vi "spotfindsettingsIngoHeucke.vi"(7 "Enum":T3(ring)=enum."change", 9 "already x spots found":i16=46, 11 "notes 2":refnum<vi>) -> (0 "settings":string="\n43 spot(s) found\nclose filter:  TRUE\nconnectivity 4/8: TRUE\nthreshold (min):  25\nthreshold (max):  1000\nselection values:\nParameter: Area (pixels)\n\t lower value: 16.00\n\t upper value: 245.00\n\t include: TRUE\nParameter: Heywood circularity factor\n\t lower value: 0.95\n\t upper value: 1.53\n\t include: TRUE\n", 2 "spotfinding settings":T2={"show all"=FALSE, "threshold/morph"=FALSE, "particle filter"=FALSE, "spot marks"=FALSE, "close filter"=TRUE, "connectivity 4/8"=TRUE, "range"={"Lower value"=25.0, "Upper value"=1000.0}, "PSF-size"=5, "Parameters"=[{"Parameter"=enum."Area (pixels)", "Lower Value"=16.0, "Upper Value"=245.0, "Interval"=TRUE}, {"Parameter"=enum."Heywood circularity factor", "Lower Value"=0.95, "Upper Value"=1.53, "Interval"=TRUE}]} {"range"."Upper value" format="%.2f"; "range"."Lower value" format="%.2f"; "Parameters"."Upper Value" format="%.2f"; "Parameters"."Lower Value" format="%.2f"}, 4 "coordinates":i32[][](array[numeric])=[[93, 0, 103, 10], [389, 8, 399, 18], [260, 10, 270, 20], [132, 13, 142, 23], [298, 19, 308, 29], [338, 32, 348, 42], [210, 38, 220, 48], [81, 41, 91, 51], [377, 45, 387, 55], [249, 50, 259, 60], [290, 60, 300, 70], [329, 74, 339, 84], [237, 89, 247, 99], [315, 110, 325, 120], [188, 117, 198, 127], [355, 124, 365, 134], [225, 128, 235, 138], [98, 128, 108, 138], [137, 143, 147, 153], [177, 156, 187, 166], [49, 160, 59, 170], [254, 179, 264, 189], [126, 183, 136, 193], [293, 190, 303, 200], [332, 201, 342, 211], [203, 207, 213, 217], [242, 217, 252, 227], [115, 223, 125, 233], [283, 231, 293, 241], [25, 238, 35, 248], [193, 246, 203, 256], [-4, 267, 6, 277], [349, 295, 359, 305], [172, 324, 182, 334], [339, 333, 349, 343], [81, 342, 91, 352], [378, 346, 388, 356], [327, 373, 337, 383], [69, 382, 79, 392], [366, 385, 376, 395], [393, 387, 403, 397], [238, 389, 248, 399], [108, 392, 118, 402]])   [LabVIEW 2009]
uses:
  spotfindersettings.ctl
panel:
  in  "range":cluster{"min.":i32, "max.":i32}={"min."=25, "max."=1000}
  out "Number of Particles":i32=43
  in  "UPDATE":bool
  in  "Selection Values":T1(array[cluster])=[{"Parameter"=enum."Area (pixels)", "Lower Value"=16.0, "Upper Value"=245.0, "Interval"=TRUE}, {"Parameter"=enum."Heywood circularity factor", "Lower Value"=0.95, "Upper Value"=1.53, "Interval"=TRUE}] {"Upper Value" format="%.2f"; "Lower Value" format="%.2f"}
  in  "scroll":u32 max=2
  in  "notes":string="file: 3.xml\r\n5/26/2011 4:32:28 PM\r\n\r\n45 spot(s) found\r\nclose filter:  TRUE\r\nconnectivity 4/8: TRUE\r\nthreshold (min):  22\r\nthreshold (max):  1000\r\nselection values:\r\nParameter: Area (pixels)\r\n\t lower value: 15.00\r\n\t upper value: 320.00\r\n\t include: TRUE\r\nParameter: Heywood circularity factor\r\n\t lower value: 0.95\r\n\t upper value: 1.61\r\n\t include: TRUE\r\n\r\nauto spot pick result spots (01 to 45) and decays stored in IMAGE PATH\r\n\r\n\r\nfile: 3.xml\r\n14.06.2011 16:14:29\r\n"
  in  "spot marks":bool
  in  "particle filter":bool
  in  "threshold/morph":bool
  in  "show all":bool
  in  "PSF-size":i32=5
  in  "connectivity 4/8":bool=TRUE
  in  "close filter":bool=TRUE
  in  "add button":bool
  in  "delete button":bool
  in  "delete element":i32 min=0 max=2
  in  "stop":bool
  # "Selection Values"
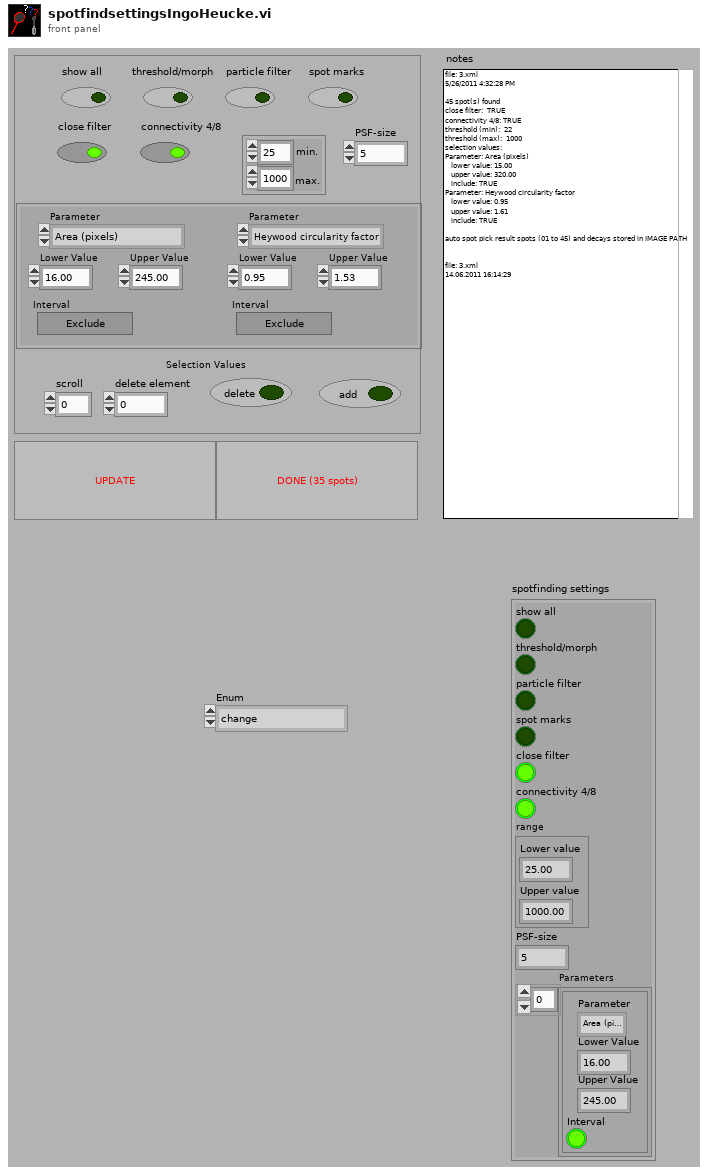
[diagram p1: front panel]
types:
  T1 = cluster{"Parameter":enum32{"Area (pixels)", "Area (calibrated)", "Number of holes", "Holes area (pixels)", "Total area (pixels)", "Scanned area (pixels)", "Ratio Area/Scanned area (%)", "Ratio Area/Total area (%)", "Center of mass (X)", "Center of mass (Y)", "Left column (X)", "Upper row (Y)", "Right column (X)", "Lower row (Y)", "Width (pixels)", "Height (pixels)", "Longest segment length", "Longest segment left column (X)", "Longest segment top row  (Y)", "Perimeter", "Holes perimeter", "SumX", "SumY", "SumXX", "SumYY", "SumXY", "Corrected projection X", "Corrected projection Y", "Moment of inertia Ixx", "Moment of inertia Iyy", "Moment of inertia Ixy", "Mean chord X", "Mean chord Y", "Max intercept", "Mean intercept perpendicular", "Particle orientation", "Equivalent ellipse minor axis", "Ellipse major axis", "Ellipse minor axis", "Ratio of equivalent ellipse axis", "Rectangle big side", "Rectangle small side", "Ratio of equivalent rectangle sides", "Elongation factor", "Compactness factor", "Heywood circularity factor", "Type factor", "Hydraulic radius", "Waddel disk diameter", "Diagonal"}, "Lower Value":sgl, "Upper Value":sgl, "Interval":bool}[]
  T2 = typedef "spotfindersettings.ctl" = cluster{"show all":bool, "threshold/morph":bool, "particle filter":bool, "spot marks":bool, "close filter":bool, "connectivity 4/8":bool, "range":cluster{"Lower value":sgl, "Upper value":sgl}, "PSF-size":i32, "Parameters":cluster{"Parameter":enum32{"Area (pixels)", "Area (calibrated)", "Number of holes", "Holes area (pixels)", "Total area (pixels)", "Scanned area (pixels)", "Ratio Area/Scanned area (%)", "Ratio Area/Total area (%)", "Center of mass (X)", "Center of mass (Y)", "Left column (X)", "Upper row (Y)", "Right column (X)", "Lower row (Y)", "Width (pixels)", "Height (pixels)", "Longest segment length", "Longest segment left column (X)", "Longest segment top row  (Y)", "Perimeter", "Holes perimeter", "SumX", "SumY", "SumXX", "SumYY", "SumXY", "Corrected projection X", "Corrected projection Y", "Moment of inertia Ixx", "Moment of inertia Iyy", "Moment of inertia Ixy", "Mean chord X", "Mean chord Y", "Max intercept", "Mean intercept perpendicular", "Particle orientation", "Equivalent ellipse minor axis", "Ellipse major axis", "Ellipse minor axis", "Ratio of equivalent ellipse axis", "Rectangle big side", "Rectangle small side", "Ratio of equivalent rectangle sides", "Elongation factor", "Compactness factor", "Heywood circularity factor", "Type factor", "Hydraulic radius", "Waddel disk diameter", "Diagonal"}, "Lower Value":sgl, "Upper Value":sgl, "Interval":bool}[]}
  T3 = enum16{"Display", "change", "get", "save", "create text", "load", "Get Refnum"}
  T4 = cluster{"show all":bool, "threshold/morph":bool, "particle filter":bool, "spot marks":bool, "close filter":bool, "connectivity 4/8":bool, "range":cluster{"Lower value":sgl, "Upper value":sgl}, "PSF-size":i32, "Parameters":cluster{"Parameter":enum32{"Area (pixels)", "Area (calibrated)", "Number of holes", "Holes area (pixels)", "Total area (pixels)", "Scanned area (pixels)", "Ratio Area/Scanned area (%)", "Ratio Area/Total area (%)", "Center of mass (X)", "Center of mass (Y)", "Left column (X)", "Upper row (Y)", "Right column (X)", "Lower row (Y)", "Width (pixels)", "Height (pixels)", "Longest segment length", "Longest segment left column (X)", "Longest segment top row  (Y)", "Perimeter", "Holes perimeter", "SumX", "SumY", "SumXX", "SumYY", "SumXY", "Corrected projection X", "Corrected projection Y", "Moment of inertia Ixx", "Moment of inertia Iyy", "Moment of inertia Ixy", "Mean chord X", "Mean chord Y", "Max intercept", "Mean intercept perpendicular", "Particle orientation", "Equivalent ellipse minor axis", "Ellipse major axis", "Ellipse minor axis", "Ratio of equivalent ellipse axis", "Rectangle big side", "Rectangle small side", "Ratio of equivalent rectangle sides", "Elongation factor", "Compactness factor", "Heywood circularity factor", "Type factor", "Hydraulic radius", "Waddel disk diameter", "Diagonal"}, "Lower Value":sgl, "Upper Value":sgl, "Interval":bool}[]}
  T5 = enum16{"Ini", "Get", "Set", "Refresh", "dump", "move", "name"}
  T6 = typedef "IMAQ Image.ctl" = refnum<image>
  T7 = enum32{"Area (pixels)", "Area (calibrated)", "Number of holes", "Holes area (pixels)", "Total area (pixels)", "Scanned area (pixels)", "Ratio Area/Scanned area (%)", "Ratio Area/Total area (%)", "Center of mass (X)", "Center of mass (Y)", "Left column (X)", "Upper row (Y)", "Right column (X)", "Lower row (Y)", "Width (pixels)", "Height (pixels)", "Longest segment length", "Longest segment left column (X)", "Longest segment top row  (Y)", "Perimeter", "Holes perimeter", "SumX", "SumY", "SumXX", "SumYY", "SumXY", "Corrected projection X", "Corrected projection Y", "Moment of inertia Ixx", "Moment of inertia Iyy", "Moment of inertia Ixy", "Mean chord X", "Mean chord Y", "Max intercept", "Mean intercept perpendicular", "Particle orientation", "Equivalent ellipse minor axis", "Ellipse major axis", "Ellipse minor axis", "Ratio of equivalent ellipse axis", "Rectangle big side", "Rectangle small side", "Ratio of equivalent rectangle sides", "Elongation factor", "Compactness factor", "Heywood circularity factor", "Type factor", "Hydraulic radius", "Waddel disk diameter", "Diagonal"}
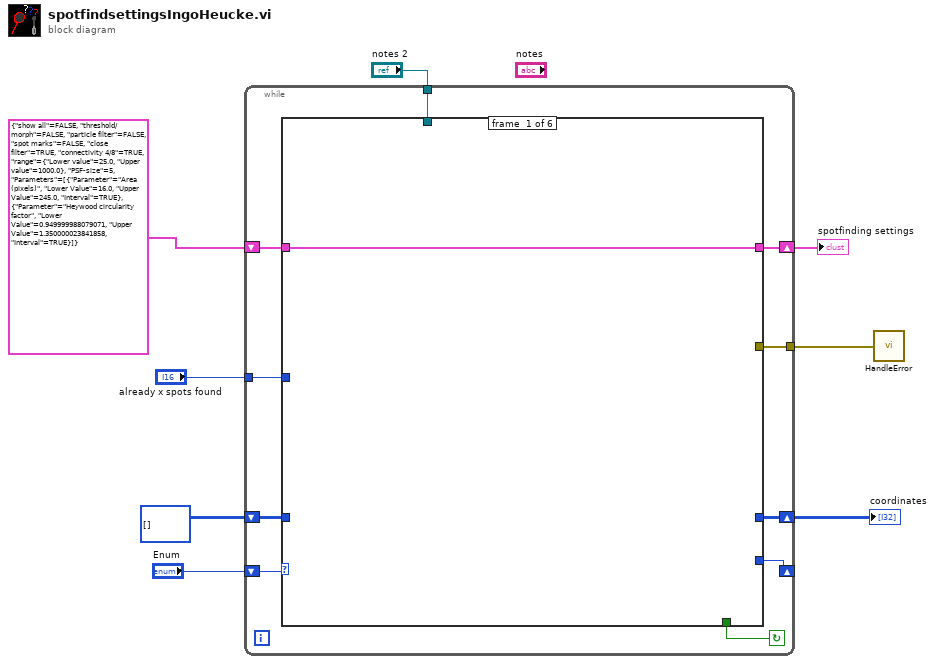
[diagram p0: block diagram]
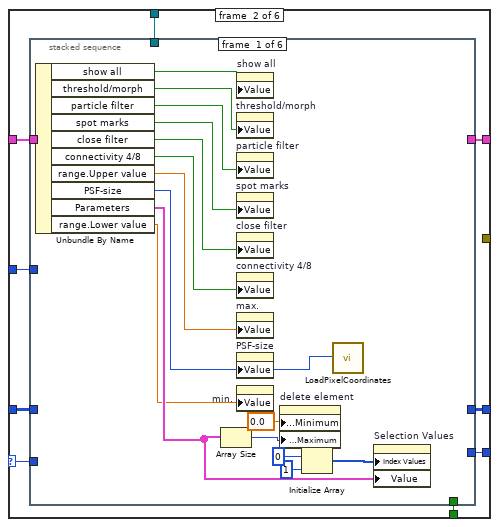
[diagram p2: hidden frame]
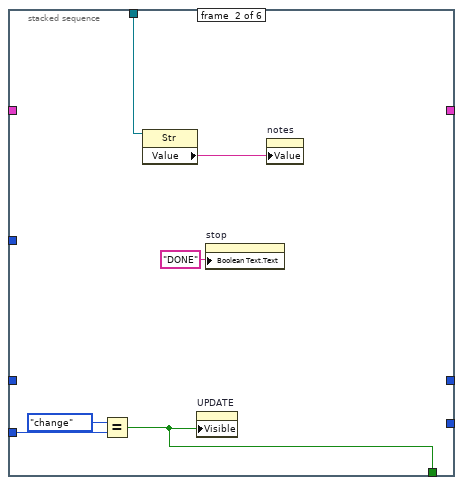
[diagram p3: hidden frame]
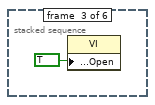
[diagram p4: hidden frame]
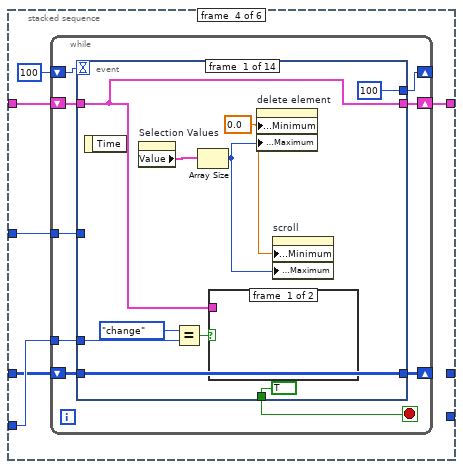
[diagram p5: hidden frame]
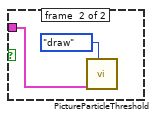
[diagram p6: hidden frame]
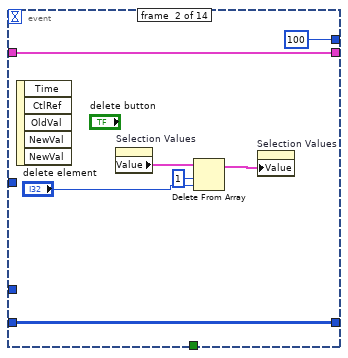
[diagram p7: hidden frame]
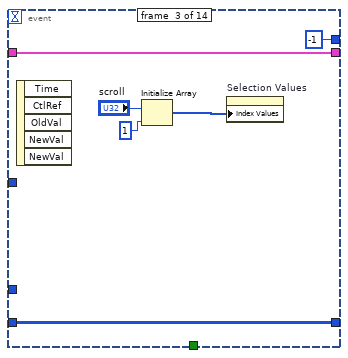
[diagram p8: hidden frame]
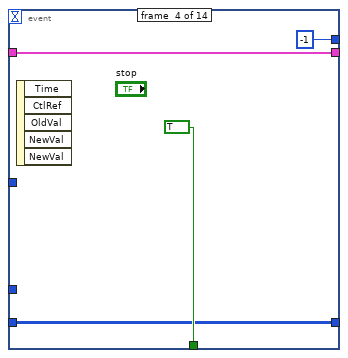
[diagram p9: hidden frame]
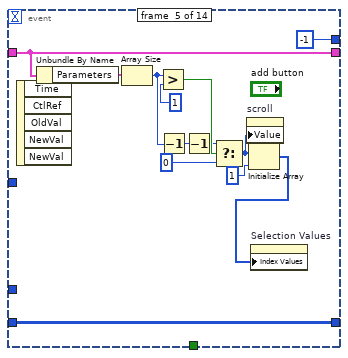
[diagram p10: hidden frame]
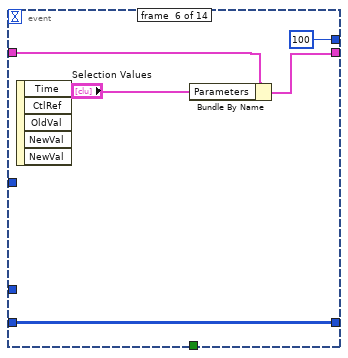
[diagram p11: hidden frame]
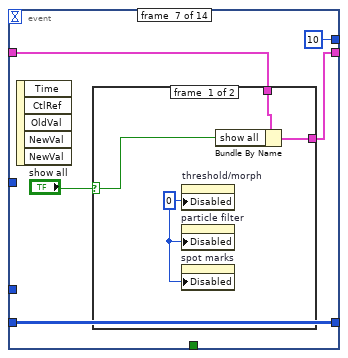
[diagram p12: hidden frame]
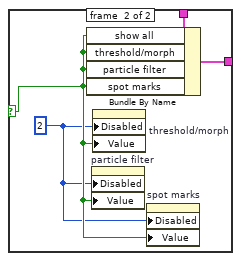
[diagram p13: hidden frame]
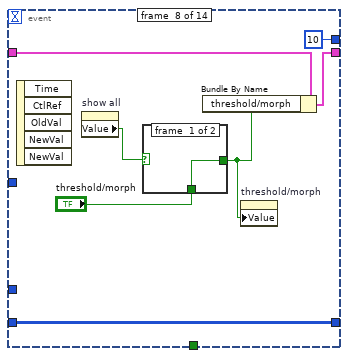
[diagram p14: hidden frame]
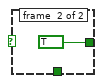
[diagram p15: hidden frame]
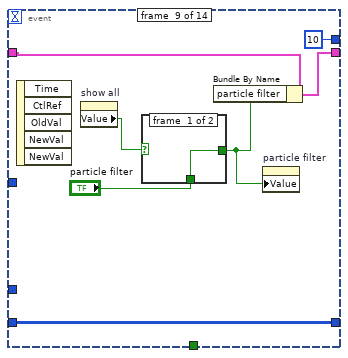
[diagram p16: hidden frame]
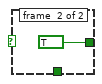
[diagram p17: hidden frame]
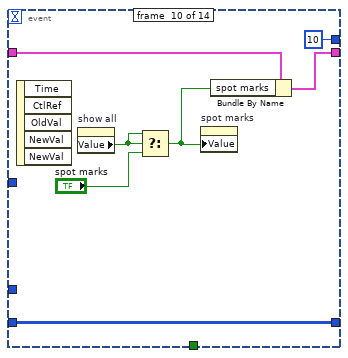
[diagram p18: hidden frame]
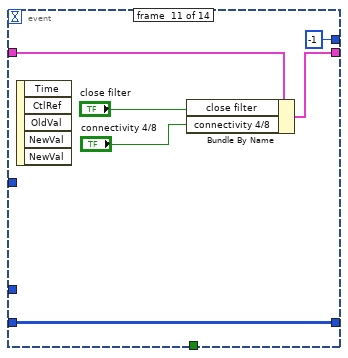
[diagram p19: hidden frame]
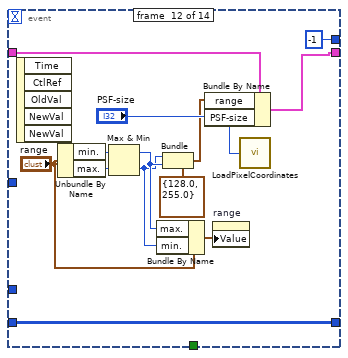
[diagram p20: hidden frame]
diagram:
  n1 = while {
    shift-right: [w9] -> w3
    shift-left: T4 {"show all"=FALSE, "threshold/morph"=FALSE, "particle filter"=FALSE, "spot marks"=FALSE, "close filter"=TRUE, "connectivity 4/8"=TRUE, "range"={"Lower value"=25.0, "Upper value"=1000.0}, "PSF-size"=5, "Parameters"=[{"Parameter"=enum."Area (pixels)", "Lower Value"=16.0, "Upper Value"=245.0, "Interval"=TRUE}, {"Parameter"=enum."Heywood circularity factor", "Lower Value"=0.95, "Upper Value"=1.35, "Interval"=TRUE}]} ("Value") -> [w10]
    tunnel: [w18] -> w2
    tunnel: "notes 2" -> [w17]
    tunnel: "already x spots found" -> [w16]
    shift-right: [w13] -> _
    shift-left: "Enum" -> [w14]
    shift-right: [w11] -> w4
    shift-left: i32[][] [] ("coordinates") -> [w12]
    stop <- w15 continue-if-true
    n2 = case shown="\"Display\", \"change\"" w14 {
      selector: w14 -> [_ w23 _ _ _ _]
      tunnel: w10 -> [w19 w28 w200 w233 w239 _]
      tunnel: [_ _ _ _ w241 _] -> w18
      tunnel: w17 -> [_ w27 _ _ _ _]
      tunnel: w16 -> [_ w26 _ _ _ _]
      tunnel: [_ w25 _ _ _ _] -> w15
      tunnel: [_ w24 _ _ _ _] -> w13
      tunnel: [_ w20 w201 _ _ _] -> w11
      tunnel: w12 -> [_ w22 w201 _ _ _]
      tunnel: [w19 w21 w200 w234 w239 w246] -> w9
      frame #0 {
      }
      frame #1 {
        n3 = stacked-sequence {
          tunnel: w28 -> [w42 _ _ w56 w186 _]
          tunnel: [_ _ _ w55 _ _] -> w21
          tunnel: w27 -> [_ w50 _ _ _ w197]
          tunnel: w26 -> [_ _ _ w54 w185 _]
          tunnel: [_ w46 _ _ _ _] -> w25
          tunnel: [_ _ _ _ _ T3."create text" ("Enum")] -> w24
          tunnel: w23 -> [_ w48 _ w53 _ _]
          tunnel: w22 -> [_ _ _ w52 _ _]
          tunnel: [_ _ _ _ w183 _] -> w20
          frame #0 {
            n4 = Unbundle By Name(w42) -> ("show all"=w41:bool, "threshold/morph"=w40:bool, "particle filter"=w39:bool, "spot marks"=w38:bool, "close filter"=w37:bool, "connectivity 4/8"=w36:bool, "range.Upper value"=w35:sgl, "PSF-size"=w34:i32, "Parameters"=w30:T1, "range.Lower value"=w29:sgl)
            n5 = Array Size(array=w30) -> (size(s)=w43:i32)
            n6 = property on="show all" class="Bool (strict)"("Value"=w41) -> ()  [unwired: 2 in, 2 out]
            n7 = property on="threshold/morph" class="Bool (strict)"("Value"=w40) -> ()  [unwired: 2 in, 2 out]
            n8 = property on="particle filter" class="Bool (strict)"("Value"=w39) -> ()  [unwired: 2 in, 2 out]
            n9 = property on="spot marks" class="Bool (strict)"("Value"=w38) -> ()  [unwired: 2 in, 2 out]
            n10 = property on="close filter" class="Bool (strict)"("Value"=w37) -> ()  [unwired: 2 in, 2 out]
            n11 = property on="connectivity 4/8" class="Bool (strict)"("Value"=w36) -> ()  [unwired: 2 in, 2 out]
            n12 = property on="max." class="DigNum (strict)"("Value"=w35) -> ()  [unwired: 2 in, 2 out]
            n13 = property on="PSF-size" class="DigNum (strict)"("Value"=w34) -> ()  [unwired: 2 in, 2 out]
            n14 = property on="min." class="DigNum (strict)"("Value"=w29) -> ()  [unwired: 2 in, 2 out]
            n15 = property on="delete element" class="Digital (strict)"("Data Entry Limits:Minimum"=0.0 ("Data Range:Minimum"), "Data Entry Limits:Maximum"=w43) -> ()  [unwired: 2 in, 2 out]
            n16 = Initialize Array(u32 0 ("element"), 1 ("dimension size")) -> (w31:u32[])
            n17 = call "LoadPixelCoordinates.vi"("spotsize (radius pixel)"=w34) -> ()
            n18 = property on="Selection Values" class="Array (strict)"("Index Values"=w31, "Value"=w30) -> ()  [unwired: 2 in, 2 out]
          }
          frame #1 {
            n19 = Equal?(x=T3."change", y=w48) -> (x = y?=w46:bool)
            n20 = property class="Str"(reference=w50) -> ("Value"=w49:string)  [unwired: 1 in, 2 out]
            n21 = property on="UPDATE" class="Bool"("Visible"=w46) -> ()  [unwired: 2 in, 2 out]
            n22 = property on="stop" class="Bool"("Boolean Text.Text"="DONE") -> ()  [unwired: 2 in, 2 out]
            n23 = property on="notes" class="String"("Value"=w49) -> ()  [unwired: 2 in, 2 out]
          }
          frame #2 {
            n24 = property class="VI"("Front Panel Window:Open"=TRUE) -> ()  [unwired: 2 in, 2 out]
          }
          frame #3 {
            n25 = while {
              shift-right: [w64] -> _
              shift-left: 100 -> [w65]
              shift-right: [w62] -> w55
              shift-left: w56 -> [w63]
              tunnel: w54 -> [w61]
              tunnel: w53 -> [w60]
              shift-right: [w59] -> _
              shift-left: w52 -> [w58]
              stop <- w66 stop-if-true
              n26 = event shown="[12] \"UPDATE\": Value Change" {
                selector: _ -> [_ _ _ _ _ _ _ _ _ _ _ _ _ _]
                dyn-events: _ -> [_ _ _ _ _ _ _ _ _ _ _ _ _ _]
                timeout: w65 -> [_ _ _ _ _ _ _ _ _ _ _ _ _ _]
                tunnel: [TRUE _ _ TRUE _ _ _ _ _ _ _ _ _ TRUE] -> w66
                tunnel: [100 100 -1 -1 -1 100 10 10 10 10 -1 -1 -1 _] -> w64
                tunnel: w63 -> [w69 w82 w91 w93 w107 w110 w116 w133 w138 w151 w157 w170 w171 w180]
                tunnel: [w69 w82 w91 w93 w107 w109 w115 w132 w139 w150 w156 w169 w171 w180] -> w62
                tunnel: w61 -> [_ _ _ _ _ _ _ _ _ _ _ _ w177 _]
                tunnel: [w68 w79 w86 w92 w96 w111 w114 w127 w136 w148 w152 w166 w176 w179] -> w59
                tunnel: w60 -> [w71 _ _ _ _ _ _ _ _ _ _ _ _ _]
                tunnel: w58 -> [w68 w79 w86 w92 w96 w111 w114 w127 w136 w148 w152 w166 _ w179]
                event #0 {
                  w74 = 0.0 ("Data Range:Minimum")
                  n27 = event-data() -> ()  [unwired: 1 in, 1 out]
                  n28 = property on="Selection Values" class="Array (strict)"() -> ("Value"=w73:T1)  [unwired: 2 in, 2 out]
                  n29 = Equal?(x=T3."change", y=w71) -> (x = y?=w72:bool)
                  n30 = Array Size(array=w73) -> (size(s)=w75:i32)
                  n31 = case shown="True" w72 {
                    tunnel: w69 -> [_ w77]
                    frame #0 {
                    }
                    frame #1 {
                      n32 = call "PictureParticleThreshold.vi"("Enum"=enum16{"new", "input", "draw", "dump"}."draw", "spotfinding settings"=w77) -> ()  [unwired: 6 in, 2 out]
                    }
                  }
                  n33 = property on="delete element" class="Digital (strict)"("Data Entry Limits:Minimum"=w74, "Data Entry Limits:Maximum"=w75) -> ()  [unwired: 2 in, 2 out]
                  n34 = property on="scroll" class="DigNum (strict)"("Data Entry Limits:Minimum"=w74, "Data Entry Limits:Maximum"=w75) -> ()  [unwired: 2 in, 2 out]
                }
                event #1 {
                  n35 = event-data() -> ()  [unwired: 1 in, 5 out]
                  n36 = property on="Selection Values" class="Array (strict)"() -> ("Value"=w80:T1)  [unwired: 2 in, 2 out]
                  n37 = Delete From Array(array=w80, length=1, index="delete element") -> (array with subset deleted=w81:T1)  [unwired: 1 out]
                  n38 = property on="Selection Values" class="Array (strict)"("Value"=w81) -> ()  [unwired: 2 in, 2 out]
                }
                event #2 {
                  n39 = event-data() -> ()  [unwired: 1 in, 5 out]
                  n40 = Initialize Array("scroll", 1 ("dimension size")) -> (w87:u32[])
                  n41 = property on="Selection Values" class="Array (strict)"("Index Values"=w87) -> ()  [unwired: 2 in, 2 out]
                }
                event #3 {
                  n42 = event-data() -> ()  [unwired: 1 in, 5 out]
                }
                event #4 {
                  n43 = event-data() -> ()  [unwired: 1 in, 5 out]
                  n44 = Unbundle By Name(w107) -> ("Parameters"=w106:T1)
                  n45 = Array Size(array=w106) -> (size(s)=w102:i32)
                  n46 = Greater?(x=w102, y=1) -> (0:w104:bool)
                  n47 = Decrement(x=w102) -> (x-1=w101:i32)
                  n48 = Decrement(x=w101) -> (x-1=w100:i32)
                  n49 = Select(t=w100, s=w104, f=u32 0) -> (s? t:f=w98:u32)
                  n50 = property on="scroll" class="DigNum (strict)"("Value"=w98) -> ()  [unwired: 2 in, 2 out]
                  n51 = Initialize Array(w98, 1 ("dimension size")) -> (w97:u32[])
                  n52 = property on="Selection Values" class="Array (strict)"("Index Values"=w97) -> ()  [unwired: 2 in, 2 out]
                }
                event #5 {
                  n53 = event-data() -> ()  [unwired: 1 in, 5 out]
                  n54 = Bundle By Name(cluster=w110, "Parameters"="Selection Values") -> (w109:T4)
                }
                event #6 {
                  n55 = event-data() -> ()  [unwired: 1 in, 5 out]
                  n56 = case shown="True" "show all" {
                    selector: "show all" -> [w120 w124]
                    tunnel: w116 -> [w122 w126]
                    tunnel: [w121 w125] -> w115
                    frame #0 {
                      w119 = u8 0 ("Disabled")
                      n57 = property on="threshold/morph" class="Bool (strict)"("Disabled"=w119) -> ()  [unwired: 2 in, 2 out]
                      n58 = property on="particle filter" class="Bool (strict)"("Disabled"=w119) -> ()  [unwired: 2 in, 2 out]
                      n59 = property on="spot marks" class="Bool (strict)"("Disabled"=w119) -> ()  [unwired: 2 in, 2 out]
                      n60 = Bundle By Name(cluster=w122, "show all"=w120) -> (w121:T4)
                    }
                    frame #1 {
                      w123 = 2
                      n61 = Bundle By Name(cluster=w126, "show all"=w124, "threshold/morph"=w124, "particle filter"=w124, "spot marks"=w124) -> (w125:T4)
                      n62 = property on="particle filter" class="Bool (strict)"("Disabled"=w123, "Value"=w124) -> ()  [unwired: 2 in, 2 out]
                      n63 = property on="threshold/morph" class="Bool (strict)"("Disabled"=w123, "Value"=w124) -> ()  [unwired: 2 in, 2 out]
                      n64 = property on="spot marks" class="Bool (strict)"("Disabled"=w123, "Value"=w124) -> ()  [unwired: 2 in, 2 out]
                    }
                  }
                }
                event #7 {
                  n65 = event-data() -> ()  [unwired: 1 in, 5 out]
                  n66 = property on="show all" class="Boolean (strict)"() -> ("Value"=w131:bool)  [unwired: 2 in, 2 out]
                  n67 = case shown="True" w131 {
                    tunnel: [w134 TRUE] -> w129
                    tunnel: "threshold/morph" -> [w134 _]
                    frame #0 {
                    }
                    frame #1 {
                    }
                  }
                  n68 = Bundle By Name(cluster=w133, "threshold/morph"=w129) -> (w132:T4)
                  n69 = property on="threshold/morph" class="Boolean (strict)"("Value"=w129) -> ()  [unwired: 2 in, 2 out]
                }
                event #8 {
                  n70 = event-data() -> ()  [unwired: 1 in, 5 out]
                  n71 = property on="show all" class="Boolean (strict)"() -> ("Value"=w142:bool)  [unwired: 2 in, 2 out]
                  n72 = case shown="True" w142 {
                    tunnel: [w143 TRUE] -> w140
                    tunnel: "particle filter" -> [w143 _]
                    frame #0 {
                    }
                    frame #1 {
                    }
                  }
                  n73 = Bundle By Name(cluster=w138, "particle filter"=w140) -> (w139:T4)
                  n74 = property on="particle filter" class="Boolean (strict)"("Value"=w140) -> ()  [unwired: 2 in, 2 out]
                }
                event #9 {
                  n75 = event-data() -> ()  [unwired: 1 in, 5 out]
                  n76 = property on="show all" class="Boolean (strict)"() -> ("Value"=w147:bool)  [unwired: 2 in, 2 out]
                  n77 = Select(t=w147, s=w147, f="spot marks") -> (s? t:f=w145:bool)
                  n78 = property on="spot marks" class="Bool (strict)"("Value"=w145) -> ()  [unwired: 2 in, 2 out]
                  n79 = Bundle By Name(cluster=w151, "spot marks"=w145) -> (w150:T4)
                }
                event #10 {
                  n80 = event-data() -> ()  [unwired: 1 in, 5 out]
                  n81 = Bundle By Name(cluster=w157, "close filter"="close filter", "connectivity 4/8"="connectivity 4/8") -> (w156:T4)
                }
                event #11 {
                  n82 = event-data() -> ()  [unwired: 1 in, 5 out]
                  n83 = Unbundle By Name("range") -> ("min."=w163:i32, "max."=w162:i32)
                  n84 = Max & Min(x=w163, y=w162) -> (max(x,y)=w160:i32, min(x,y)=w159:i32)
                  n85 = Bundle By Name(cluster="range", "max."=w160, "min."=w159) -> (w158:cluster{"min.":i32, "max.":i32})
                  n86 = Bundle(cluster=cluster{"Lower value":sgl, "Upper value":sgl} {"Lower value"=128.0, "Upper value"=255.0} ("Range"), "Lower value"=w159, "Upper value"=w160) -> (w165:cluster{"Lower value":sgl, "Upper value":sgl})
                  n87 = Bundle By Name(cluster=w170, "range"=w165, "PSF-size"="PSF-size") -> (w169:T4)
                  n88 = property on="range" class="Cluster (strict)"("Value"=w158) -> ()  [unwired: 2 in, 2 out]
                  n89 = call "LoadPixelCoordinates.vi"("spotsize (radius pixel)"="PSF-size") -> ()
                }
                event #12 {
                  n90 = event-data() -> ()  [unwired: 1 in, 5 out]
                  n91 = call "UpdateAutoSpotFoundAfterSettingsChange.vi"("spotfinding settings"=w171, "already x spots found"=w177) -> ("coordinates"=w176:i32[][], "Number of Particles"=w174:i32)
                  "Number of Particles" <- w174
                  n92 = Format Into String(format string="(%d spots)", initial string="DONE ", w174) -> (resulting string=w175:string)  [unwired: 1 in, 1 out]
                  n93 = property on="stop" class="Bool"("Boolean Text.Text"=w175) -> ()  [unwired: 2 in, 2 out]
                }
                event #13 {
                  n94 = event-data() -> ()  [unwired: 1 in, 3 out]
                  n95 = event-data("Discard?"=FALSE) -> ()  [unwired: 1 in, 1 out]
                }
              }
            }
          }
          frame #4 {
            n96 = call "UpdateAutoSpotFoundAfterSettingsChange.vi"("spotfinding settings"=w186, "already x spots found"=w185) -> ("coordinates"=w183:i32[][], "Number of Particles"=w184:i32)
            n97 = Format Into String(format string="(%d spots)", initial string="DONE ", w184) -> (resulting string=w189:string)  [unwired: 1 in, 1 out]
            n98 = local write "Number of Particles"(w184) -> ()
            n99 = property on="stop" class="Bool"("Boolean Text.Text"=w189) -> ()  [unwired: 2 in, 2 out]
          }
          frame #5 {
            n100 = call "FilePathGlobal.vi"("set?"=FALSE) -> ("Image Path 2"=w192:path)  [unwired: 1 in, 2 out]
            n101 = property on="notes" class="Str"() -> ("Value"=w198:string)  [unwired: 2 in, 2 out]
            n102 = property class="VI"("Front Panel Window:Open"=FALSE) -> ()  [unwired: 2 in, 2 out]
            n103 = call "Intensityduplex.vi"("Enum"=T5."Get") -> ("Image Duplicate (out)"=w194:T6)  [unwired: 4 in, 1 out]
            n104 = call "changefilename.vi"("suffix"="_spots.png", "path in"=w192) -> ("path out"=w190:path)  [unwired: 1 out]
            n105 = property on="Property Node" class="Str"(reference=w197, "Value"=w198) -> ()  [unwired: 1 in, 2 out]
            n106 = call-poly "IMAQ Write File 2"("File Path"=w190, "Image"=w194) -> ()  [unwired: 8 in, 2 out]
          }
        }
      }
      frame #2 {
        n107 = stacked-sequence {
          seq-local: [w208 _] -> [_ w223]
          tunnel: w200 -> [w212 w221]
          frame #0 {
            n108 = Unbundle By Name(w212) -> ("close filter"=w211:bool, "connectivity 4/8"=w210:bool, "range.Lower value"=w209:sgl, "range.Upper value"=w202:sgl)
            n109 = Format Into String(format string="%s %s\\n%s %s\\n%s %d\\n%s %d\\n", "close filter: ", w211, "connectivity 4/8:" ("input 3"), w210, "threshold (min): ", w209, "threshold (max): ", w202) -> (resulting string=w207:string)  [unwired: 2 in, 1 out]
            n110 = property on="Number of Particles" class="Digital (strict)"() -> ("Value"=w206:i32)  [unwired: 2 in, 2 out]
            n111 = Format Into String(format string="\\n%d\\sspot(s)\\sfound\\n", w206) -> (resulting string=w205:string)  [unwired: 2 in, 1 out]
            n112 = Concatenate Strings(w205, w207) -> (w208:string)
          }
          frame #1 {
            n113 = Unbundle By Name(w221) -> ("Parameters"=w217:T1)
            n114 = for {
              shift-right: [w230] -> w220
              shift-left: "" -> [w231]
              tunnel: w217 -> [w228] mode=indexing
              n115 = Unbundle By Name(w228) -> ("Parameter"=w227:T7, "Lower Value"=w226:sgl, "Upper Value"=w225:sgl, "Interval"=w224:bool)
              n116 = Format Into String(format string="Parameter: %s\\n\\t lower value: %.2f\\n\\t upper value: %.2f\\n\\t include: %s\\n", w227, w226, w225, w224) -> (resulting string=w232:string)  [unwired: 2 in, 1 out]
              n117 = Concatenate Strings(w231, w232) -> (w230:string)
            }
            n118 = Concatenate Strings(w223, "selection values:\n", w220) -> (→"settings":string)
          }
        }
      }
      frame #3 {
        n119 = Current VI's Path() -> (path=w238:path)
        n120 = Strip Path(path=w238) -> (stripped path=w237:path)  [unwired: 1 out]
        n121 = Build Path(base path=w237, name or relative path="autospotting.set") -> (appended path=w235:path)
        n122 = Read from Binary File(5:w233, 11:w235) -> (2:w234:T4)  [unwired: 4 in, 3 out]
      }
      frame #4 {
        n123 = Current VI's Path() -> (path=w245:path)
        n124 = Strip Path(path=w245) -> (stripped path=w244:path)  [unwired: 1 out]
        n125 = Build Path(base path=w244, name or relative path="autospotting.set") -> (appended path=w242:path)
        n126 = Write to Binary File(file (use dialog)=w242, data=w239, 5:TRUE ("prepend array or string size? (T)")) -> (error out=w241:errorcluster)  [unwired: 3 in, 2 out]
      }
      frame #5 {
        n127 = property on="spotfinding settings" class="Clust (strict)"() -> ("Value"=w246:T4)  [unwired: 2 in, 2 out]
      }
    }
  }
  "spotfinding settings" <- w3
  "coordinates" <- w4
  n128 = call "HandleError.vi"("error in (no error)"=w2) -> ()
